vi "tokens_to_expression.vi"(11 "Tokens in":string[](array[string])) -> (2 "Tokens out":string[](array[string]), 3 "Expression out":T1)   [LabVIEW 2021]
uses:
  Expression.ctl
  ExpressionType.ctl
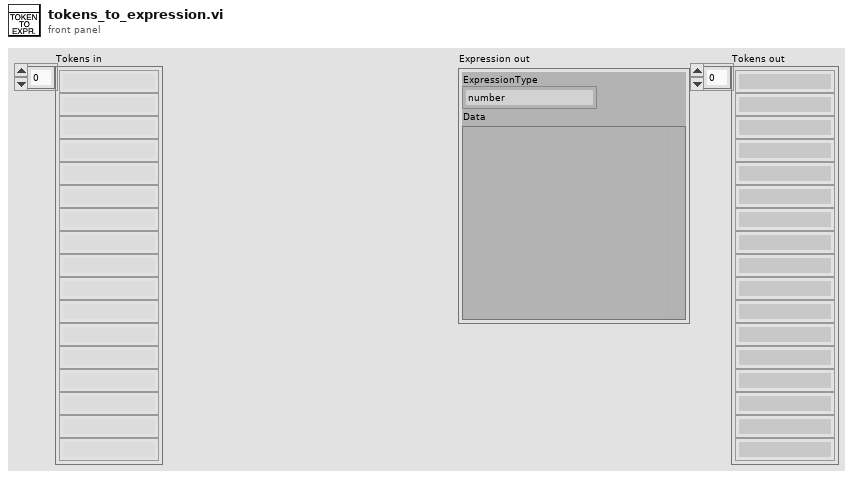
[diagram p1: front panel]
types:
  T1 = typedef "Expression.ctl" = cluster{"ExpressionType":T2, "Data":variant}
  T2 = typedef "ExpressionType.ctl" = enum16{"number", "string", "symbol", "primitive", "list", "closure", "nil", "error"}
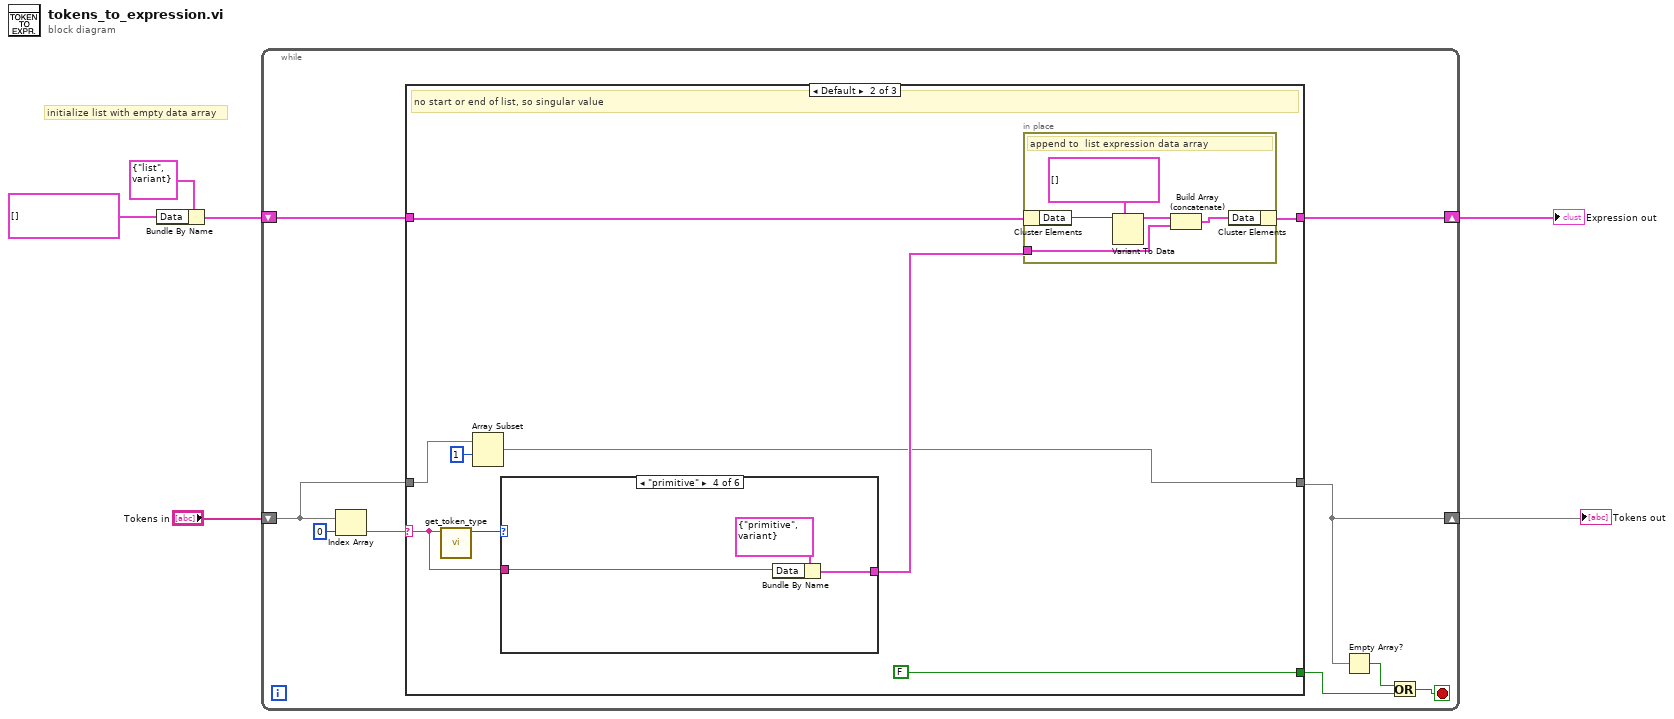
[diagram p0: block diagram]
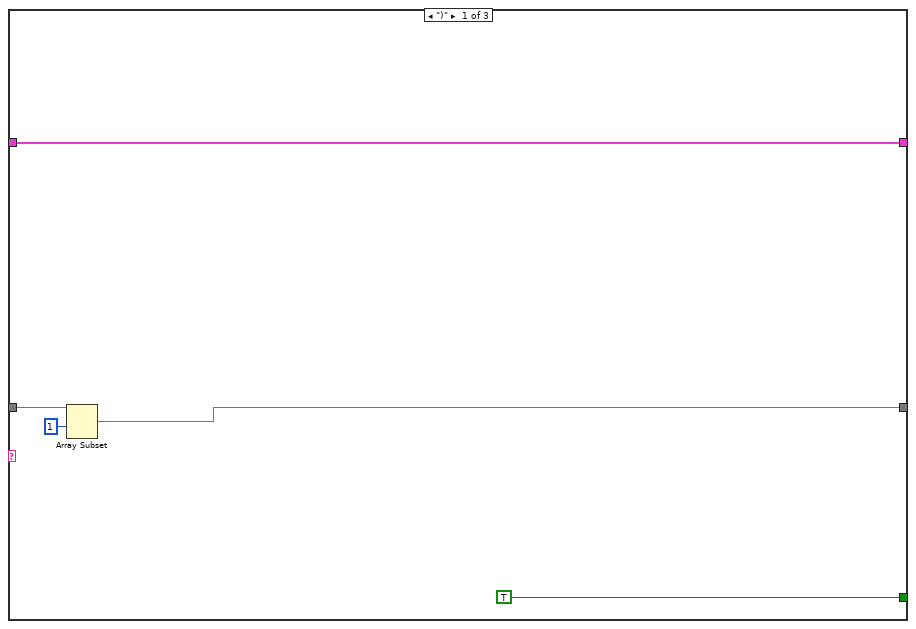
[diagram p2: hidden frame]
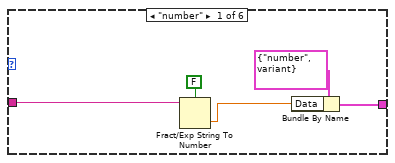
[diagram p3: hidden frame]
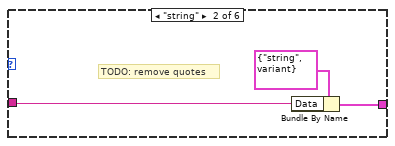
[diagram p4: hidden frame]
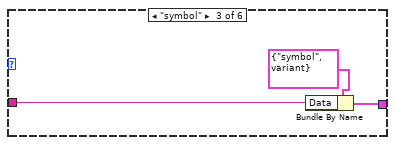
[diagram p5: hidden frame]
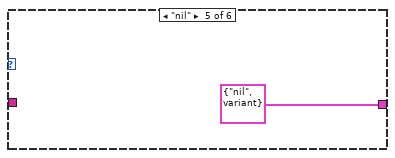
[diagram p6: hidden frame]
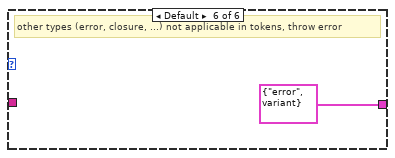
[diagram p7: hidden frame]
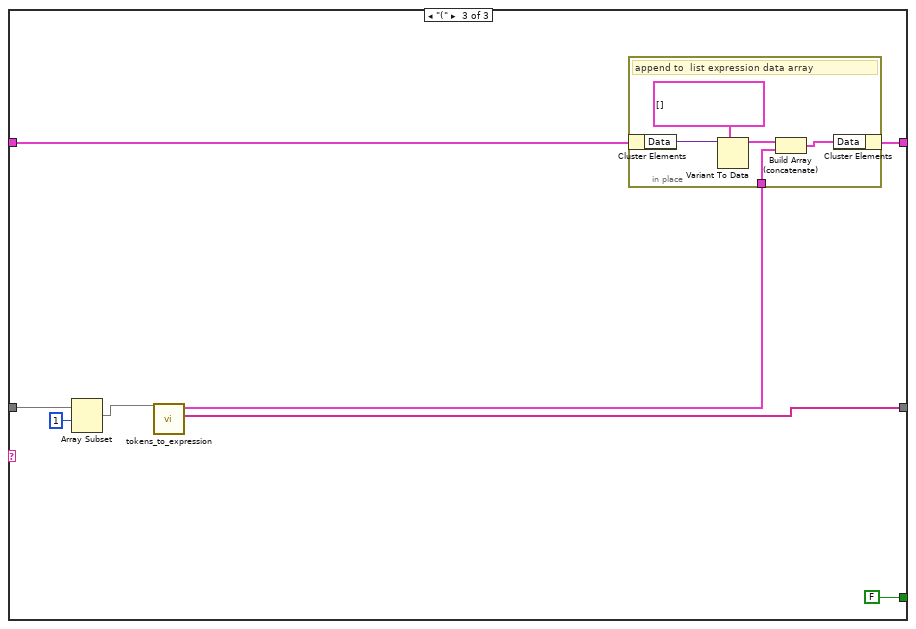
[diagram p8: hidden frame]
diagram:
  # "initialize list with empty data array"
  n1 = Bundle By Name(cluster=T1 {"ExpressionType"=enum."list", "Data"=variant} ("Expression out"), "Data"=T1[] []) -> (w1:T1)
  n2 = while {
    shift-right: [w13] -> w5
    shift-left: w1 -> [w12]
    shift-right: [w7] -> w4
    shift-left: "Tokens in" -> [w11]
    stop <- w10 stop-if-true
    n3 = Index Array(array=w11, index=0) -> (element=w15:string)
    n4 = case shown="Default" w15 {
      selector: w15 -> [_ w27 _]
      tunnel: [TRUE FALSE FALSE] -> w9
      tunnel: [w19 w26 w57] -> w13
      tunnel: w12 -> [w19 w25 w56]
      tunnel: w11 -> [w17 w22 w52]
      tunnel: [w16 w21 w54] -> w7
      frame ")" {
        n5 = Array Subset(array=w17, index=1) -> (w16:string[])  [unwired: 1 in]
      }
      frame Default {
        # "no start or end of list, so singular value"
        n6 = call "get_token_type.vi"("token"=w27) -> ("ExpressionType"=w28:T2)  [unwired: 10 in]
        n7 = Array Subset(array=w22, index=1) -> (w21:string[])  [unwired: 1 in]
        n8 = case shown="\"primitive\"" w28 {
          tunnel: w27 -> [w36 w41 w44 w47 _ _]
          tunnel: [w35 w40 w43 w46 T1 {"ExpressionType"=enum."nil", "Data"=variant} ("Expression out") T1 {"ExpressionType"=enum."error", "Data"=variant} ("Expression out")] -> w24
          frame "number" {
            n9 = Fract/Exp String To Number(use system decimal point (T)=FALSE, string=w36) -> (number=w37:dbl)  [unwired: 2 in, 1 out]
            n10 = Bundle By Name(cluster=T1 {"ExpressionType"=enum."number", "Data"=variant} ("Expression out"), "Data"=w37) -> (w35:T1)
          }
          frame "string" {
            # "TODO: remove quotes"
            n11 = Bundle By Name(cluster=T1 {"ExpressionType"=enum."string", "Data"=variant} ("Expression out"), "Data"=w41) -> (w40:T1)
          }
          frame "symbol" {
            n12 = Bundle By Name(cluster=T1 {"ExpressionType"=enum."symbol", "Data"=variant} ("Expression out"), "Data"=w44) -> (w43:T1)
          }
          frame "primitive" {
            n13 = Bundle By Name(cluster=T1 {"ExpressionType"=enum."primitive", "Data"=variant} ("Expression out"), "Data"=w47) -> (w46:T1)
          }
          frame "nil" {
          }
          frame Default {
            # "other types (error, closure, ...) not applicable in tokens, throw error"
          }
        }
        n14 = in-place {
          in-place-border: w24 -> [w30]
          # "append to  list expression data array"
          n15 = in-place-cluster #1(w25) -> ("Data"=w34:variant)
          n16 = Variant To Data(type=T1[] [], Variant=w34) -> (data=w32:T1[])  [unwired: 1 in, 1 out]
          n17 = Build Array (concatenate)(w32, w30) -> (w31:T1[])
          n18 = in-place-cluster #1("Data"=w31) -> (w26:T1)
        }
      }
      frame "(" {
        n19 = Array Subset(array=w52, index=1) -> (w51:string[])  [unwired: 1 in]
        n20 = call "tokens_to_expression.vi"("Tokens in"=w51) -> ("Tokens out"=w54:string[], "Expression out"=w55:T1)  [unwired: 9 in]
        n21 = in-place {
          in-place-border: w55 -> [w59]
          # "append to  list expression data array"
          n22 = in-place-cluster #2(w56) -> ("Data"=w63:variant)
          n23 = Variant To Data(type=T1[] [], Variant=w63) -> (data=w61:T1[])  [unwired: 1 in, 1 out]
          n24 = Build Array (concatenate)(w61, w59) -> (w60:T1[])
          n25 = in-place-cluster #2("Data"=w60) -> (w57:T1)
        }
      }
    }
    n26 = Empty Array?(array=w7) -> (empty?=w8:bool)
    n27 = Or(x=w8, y=w9) -> (x .or. y?=w10:bool)
  }
  "Expression out" <- w5
  "Tokens out" <- w4
